vi "NanotecSMCPDDriver.get standby current.vi"(0 "VISA resource name":refnum<visa-resource-name>, 1 "contollerID":i32=-1, 5 "error in (no error)":errorcluster) -> (14 "VISA resource name out":refnum<visa-resource-name>, 15 "contollerID out":i32=-1, 17 "standbyCurrent [A]":dbl, 19 "error out":errorcluster)   [LabVIEW 2014, in "NanotecSMCPDDriver.lvlib"]
doc: "Gets the phase current of the motor that will be used, when the motor is not moving."
uses:
  NanotecSMCPDDriver.lvlib
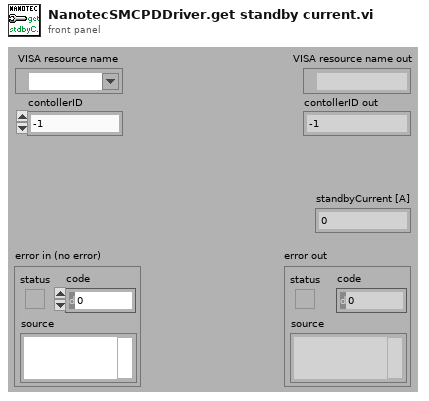
[diagram p1: front panel]
types:
  T1 = typedef "NanotecSMCPDDriver.lvlib/NanotecSMCPDDriver.hardware types.ctl" = enum16{"unknown", "PD4", "PD4Ic", "PD2Ic", "SMCI32", "SMCI47"}
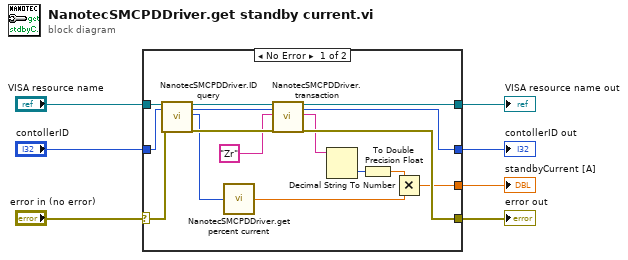
[diagram p0: block diagram]
diagram:
  n1 = case shown="No Error" "error in (no error)" {
    selector: "error in (no error)" -> [w16 w24]
    tunnel: [w22 w26] -> w7
    tunnel: [w21 w24] -> w6
    tunnel: "VISA resource name" -> [w20 w26]
    tunnel: "contollerID" -> [w19 w25]
    tunnel: [w23 w25] -> w3
    tunnel: [w8 _] -> w1
    frame No Error {
      n2 = call "NanotecSMCPDDriver.ID query.vi"("VISA resource name"=w20, "contollerID"=w19, "error in (no error)"=w16) -> ("VISA resource name out"=w17:refnum<visa-resource-name>, "contollerID out"=w18:i32, "hardwareType"=w14:T1, "error out"=w15:errorcluster)  [unwired: 12 in, 1 out]
      n3 = call "NanotecSMCPDDriver.get percent current.vi"("hardwareType"=w14) -> ("percentCurrent [A/%]"=w10:dbl)
      n4 = call "NanotecSMCPDDriver.transaction.vi"("VISAresource"=w17, "contollerID"=w18, "commandString"="Zr", "error in (no error)"=w15) -> ("VISAresource out"=w22:refnum<visa-resource-name>, "contollerID out"=w23:i32, "response"=w12:string, "error out"=w21:errorcluster)  [unwired: 10 in, 2 out]
      n5 = Decimal String To Number(string=w12) -> (number=w11:i32)  [unwired: 2 in, 1 out]
      n6 = To Double Precision Float(number=w11) -> (double precision float=w9:dbl)
      n7 = Multiply(x=w9, y=w10) -> (x*y=w8:dbl)
    }
    frame Error {
    }
  }
  "standbyCurrent [A]" <- w1
  "VISA resource name out" <- w7
  "error out" <- w6
  "contollerID out" <- w3
